vi "Servo MSMT TDSCDMA Create Evaluations.vi"(8 "error in (no error)":errorcluster, 11 "Servo MSMT in":refnum<class "Servo MSMT.lvclass">) -> (0 "error out":errorcluster, 2 "WCDMA Evaluations":T1[](array[typedef]) {"Low Limit" format="%#_13g"; "SI Scaling" items=["femto"=-15, "pico"=-12, "nano"=-9, "micro"=-6, "milli"=-3, "percent"=-2, ""=0, "kilo"=3, "mega"=6, "giga"=9, "tera"=12]}, 3 "Servo MSMT out":refnum<class "Servo MSMT.lvclass">)   [LabVIEW 2018, in "Servo MSMT.lvlib" / "Servo MSMT.lvclass"]
uses:
  Servo MSMT.lvclass
  C:/Sequence Automation/Plugins/Measurement Interface.lvlibp/Measurement Interface.lvclass
  Plugins/TestStand API Tools (TSAT).lvlibp/Evaluation Actions/Includes/Controls/TSAT Evaluation.ctl
  Plugins/TestStand API Tools (TSAT).lvlibp/Evaluation Actions/Includes/Controls/TSAT Eval SI Unit Scaling.ctl
  Plugins/TestStand API Tools (TSAT).lvlibp/Evaluation Actions/Includes/Controls/TSAT Evaluation Type.ctl
  Servo MSMT.lvclass/Servo MSMT.ctl
  Plugins/SeqAuto IEvaluation.lvlibp/SeqAuto IEvaluation.lvclass
  Protected Methods/Read DC Pins.vi
  Protected Methods/Read Servo Measurements.vi
  Plugins/SeqAuto Evaluations.lvlibp/TDSCDMA Evaluations/TDSCDMA_ACP/TDSCDMA_ACP.lvclass
  C:/Sequence Automation/Plugins/SeqAuto IEvaluation.lvlibp/SeqAuto IEvaluation.lvclass
  Plugins/SeqAuto Evaluations.lvlibp/TDSCDMA Evaluations/TDSCDMA_OBW/TDSCDMA_OBW.lvclass
  Plugins/SeqAuto Evaluations.lvlibp/TDSCDMA Evaluations/TDSCDMA_CHP/TDSCDMA_CHP.lvclass
  Plugins/SeqAuto Evaluations.lvlibp/TDSCDMA Evaluations/TDSCDMA_SEM/TDSCDMA_SEM.lvclass
  Plugins/SeqAuto Evaluations.lvlibp/Servo/Servo Gain/Servo Gain.lvclass
  Plugins/SeqAuto Evaluations.lvlibp/PA Evaluations/PAE/PAE.lvclass
  Plugins/SeqAuto Evaluations.lvlibp/TDSCDMA Evaluations/TDSCDMA_MODACC/TDSCDMA_MODACC.lvclass
  Plugins/SeqAuto Evaluations.lvlibp/DC Evaluations/DC_IDD.lvclass
  Plugins/Measurement Interface.lvlibp/Private Methods/Measurement Name/Read Measurement Name.vi
  Plugins/Measurement Interface.lvlibp/Private Methods/Measurement Parameters/Read Measurement Parameters.vi
  Plugins/String Database.lvlibp/String Database.lvclass
  Plugins/TestStand API Tools (TSAT).lvlibp/Evaluation Actions/TSAT Evaluation Actions.lvlib
  Plugins/Test Number and Bin Generator.lvlibp/Test Number and Bin Generator/Test Number and Bin Generator.lvclass
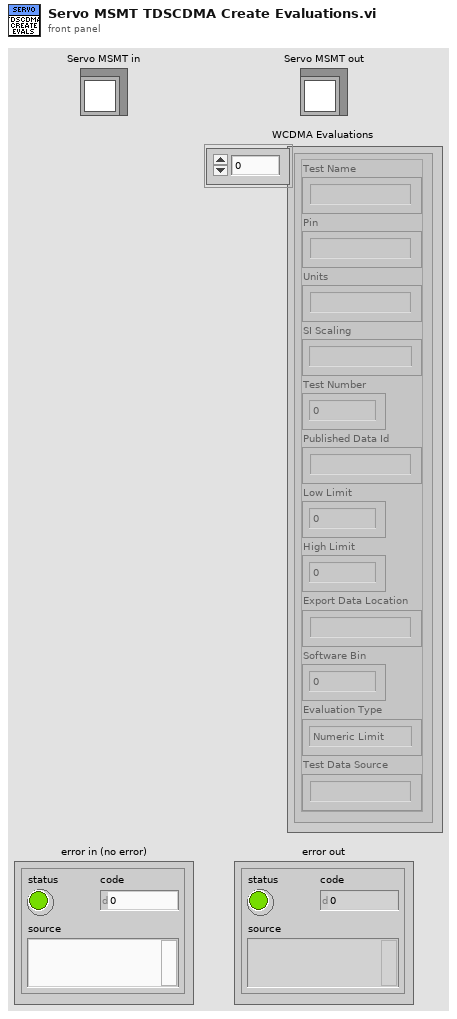
[diagram p1: front panel]
types:
  T1 = typedef "TestStand API Tools (TSAT).lvlibp/TSAT Evaluation Actions.lvlib/TSAT Evaluation.ctl" = cluster{"Test Name":string, "Pin":string, "Units":string, "SI Scaling":T2, "Test Number":i32, "Published Data Id":string, "Low Limit":dbl, "High Limit":dbl, "Export Data Location":string, "Software Bin":i64, "Evaluation Type":T3, "Test Data Source":string}
  T2 = typedef "TestStand API Tools (TSAT).lvlibp/TSAT Evaluation Actions.lvlib/TSAT Eval SI Unit Scaling.ctl" = i16
  T3 = typedef "TestStand API Tools (TSAT).lvlibp/TSAT Evaluation Actions.lvlib/TSAT Evaluation Type.ctl" = enum16{"Numeric Limit", "Pass/Fail", "None"}
  T4 = typedef "Test Number and Bin Generator.lvlibp/Test Number and Bin Generator.lvclass/Session Handle.ctl" = refnum<data-value>
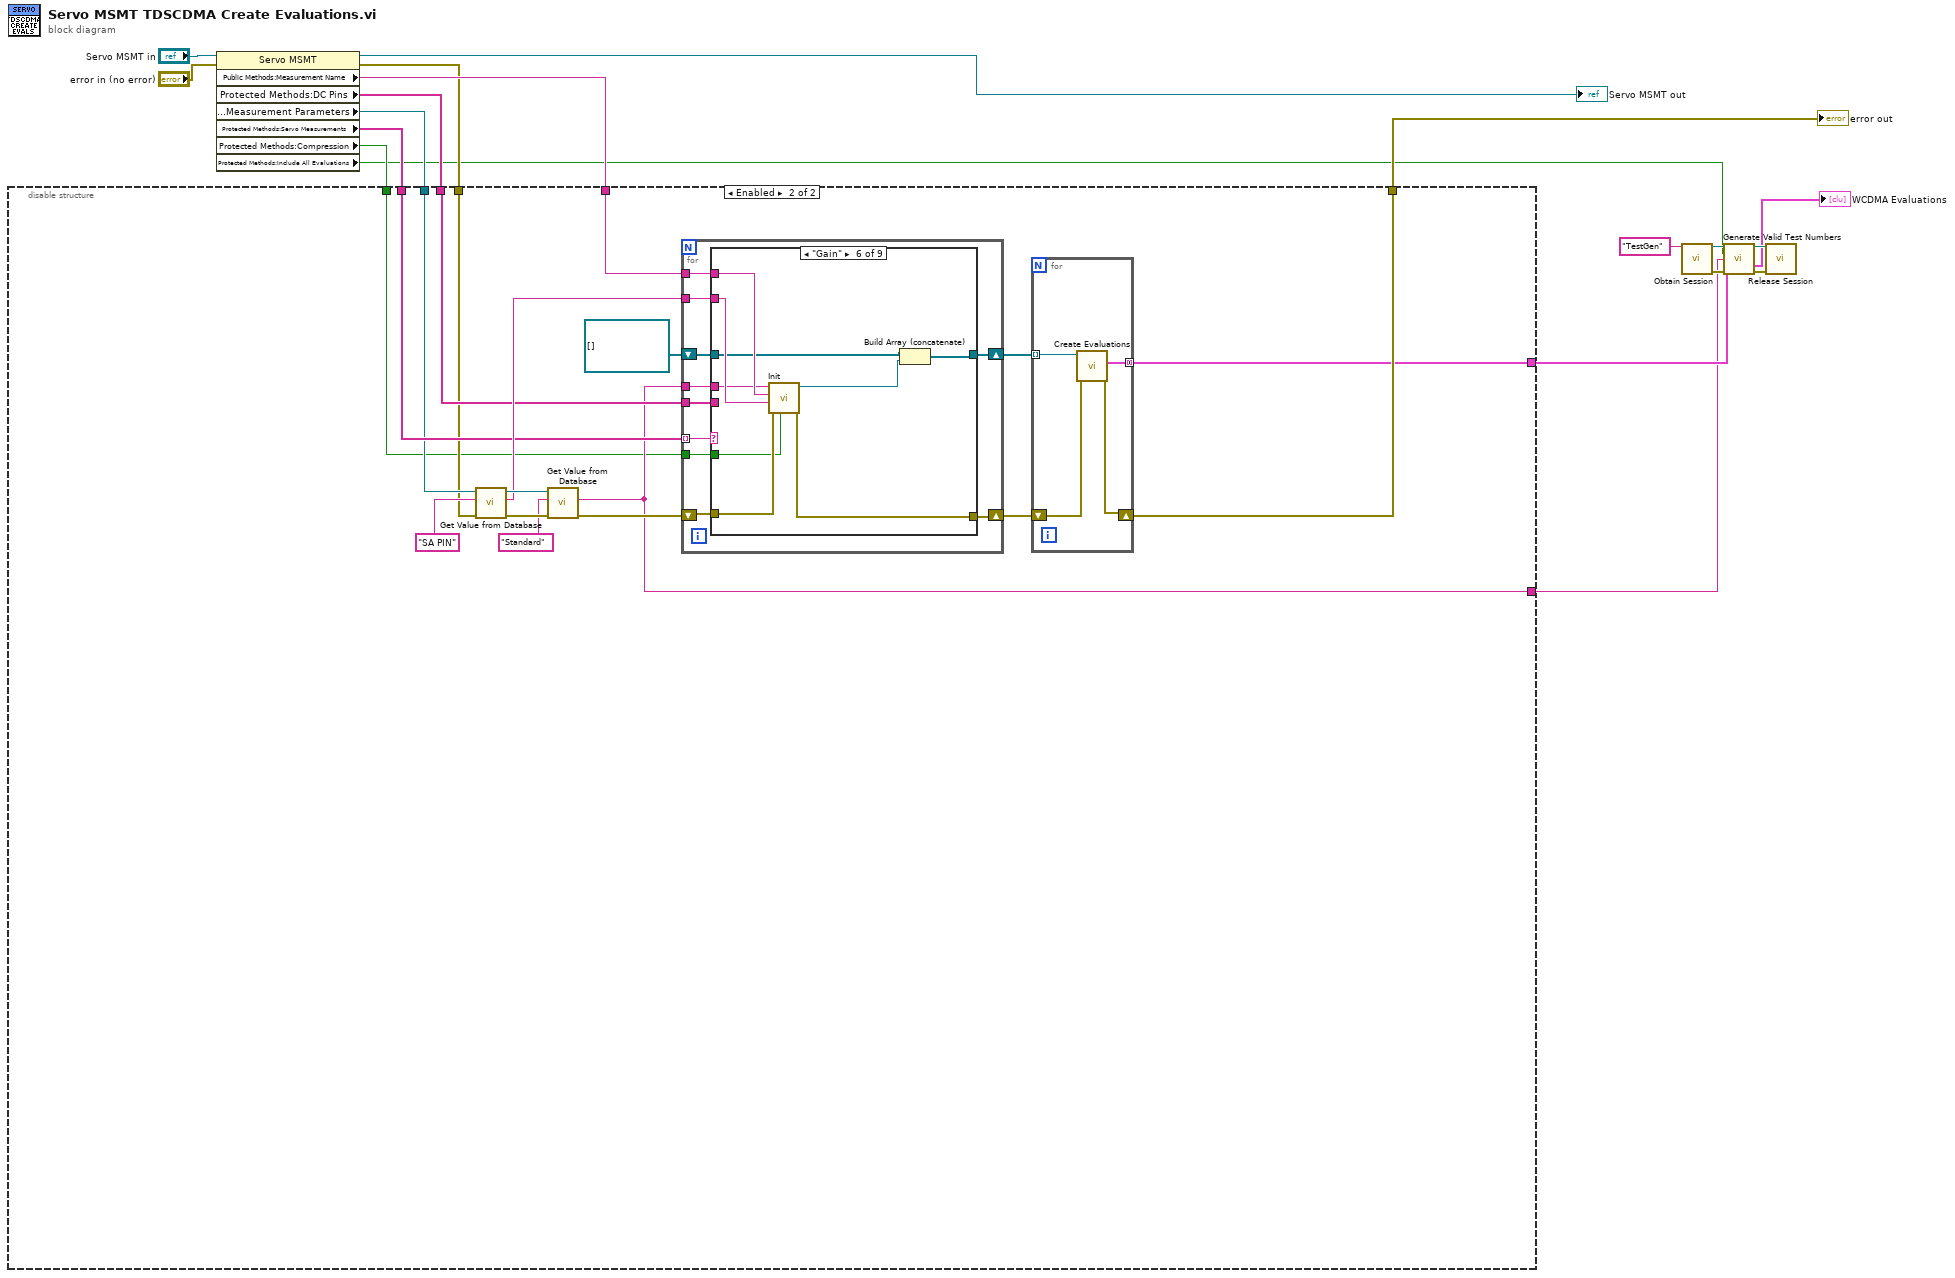
[diagram p0: block diagram]
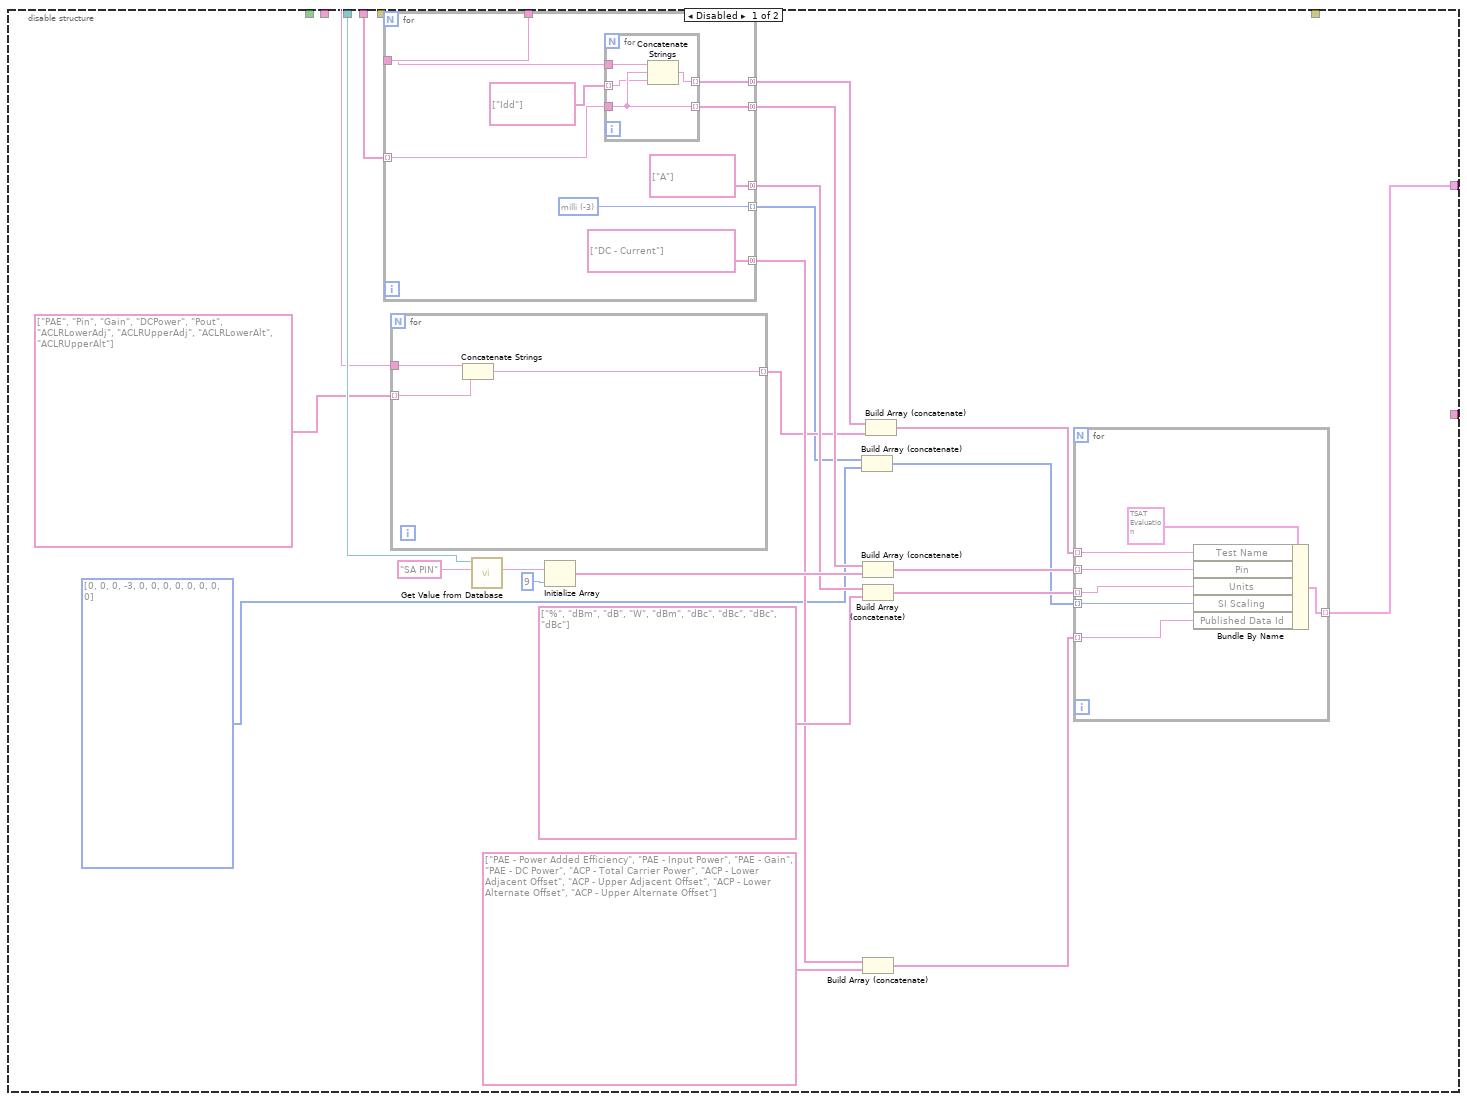
[diagram p2: hidden frame]
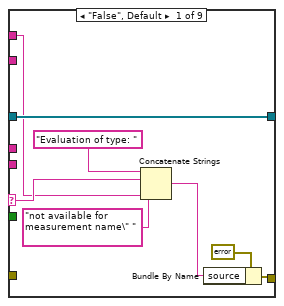
[diagram p3: hidden frame]
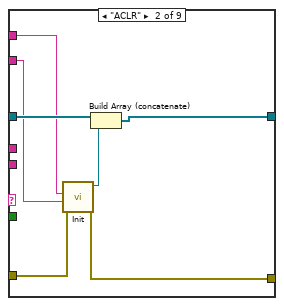
[diagram p4: hidden frame]
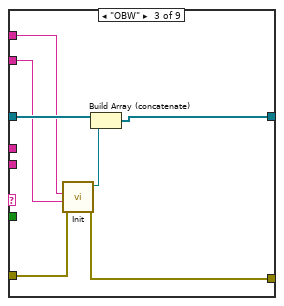
[diagram p5: hidden frame]
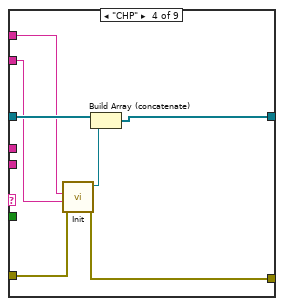
[diagram p6: hidden frame]
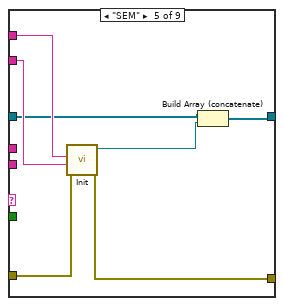
[diagram p7: hidden frame]
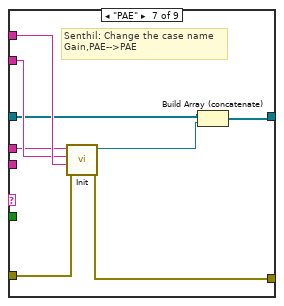
[diagram p8: hidden frame]
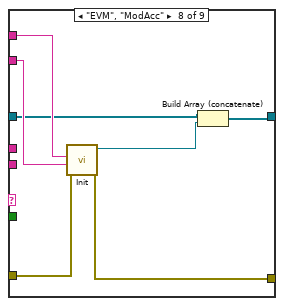
[diagram p9: hidden frame]
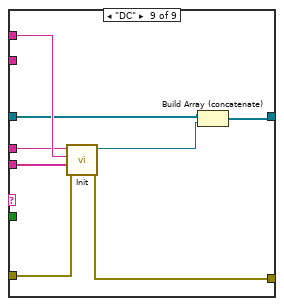
[diagram p10: hidden frame]
diagram:
  n1 = property class="Servo MSMT"(reference="Servo MSMT in", error in="error in (no error)") -> (reference out=→"Servo MSMT out":refnum<class "Servo MSMT.lvclass">, error out=w6:errorcluster, "Public Methods:Measurement Name"=w13:string, "Protected Methods:DC Pins"=w16:string[], "Protected Methods:Measurement Parameters"=w15:refnum<class "String Database.lvclass">, "Protected Methods:Servo Measurements"=w4:string[], "Protected Methods:Compression"=w2:bool, "Protected Methods:Include All Evaluations"=w1:bool)
  n2 = disable-structure shown="Enabled" {
    disable-tunnel: w16 -> [w42 w70]
    disable-tunnel: w15 -> [w40 w71]
    disable-tunnel: w13 -> [w25 w73]
    disable-tunnel: [w20 w66] -> w7
    disable-tunnel: w6 -> [_ w69]
    disable-tunnel: [_ w67] -> w5
    disable-tunnel: w4 -> [_ w72]
    disable-tunnel: [_ w68] -> w3
    disable-tunnel: w2 -> [_ w65]
    frame Disabled {
      w21 = T2[] [0, 0, 0, -3, 0, 0, 0, 0, 0, 0, 0, 0] items=["femto"=-15, "pico"=-12, "nano"=-9, "micro"=-6, "milli"=-3, "percent"=-2, ""=0, "kilo"=3, "mega"=6, "giga"=9, "tera"=12]
      n3 = for {
        tunnel: w42 -> [w50] mode=indexing
        tunnel: w25 -> [w47]
        tunnel: [w52] -> w41 mode=concatenating
        tunnel: [string[] ["A"]] -> w32 mode=concatenating
        tunnel: [w49] -> w36 mode=concatenating
        tunnel: [string[] ["DC - Current"]] -> w30 mode=concatenating
        tunnel: [w46] -> w23 mode=indexing
        w46 = T2 -3 items=["femto"=-15, "pico"=-12, "nano"=-9, "micro"=-6, "milli"=-3, "percent"=-2, ""=0, "kilo"=3, "mega"=6, "giga"=9, "tera"=12] ("SI Scaling")
        n4 = for {
          tunnel: w47 -> [w57]
          tunnel: string[] ["Idd"] -> [w54] mode=indexing
          tunnel: [w56] -> w52 mode=indexing
          tunnel: w50 -> [w55]
          tunnel: [w55] -> w49 mode=indexing
          n5 = Concatenate Strings(w57, w55, w54) -> (w56:string)
        }
      }
      n6 = for {
        tunnel: string[] ["PAE", "Pin", "Gain", "DCPower", "Pout", "ACLRLowerAdj", "ACLRUpperAdj", "ACLRLowerAlt", "ACLRUpperAlt"] -> [w44] mode=indexing
        tunnel: w25 -> [w45]
        tunnel: [w43] -> w24 mode=indexing
        n7 = Concatenate Strings(w45, w44) -> (w43:string)
      }
      n8 = call "Get Value from Database.vi"("Entry Name"="SA PIN", "Message in"=w40) -> ("Entry Value"=w37:string)  [unwired: 6 in, 3 out]
      n9 = Initialize Array(w37, 9) -> (w35:string[])
      n10 = Build Array (concatenate)(w23, w21) -> (w22:T2[])
      n11 = Build Array (concatenate)(w36, w35) -> (w34:string[])
      n12 = Build Array (concatenate)(w32, string[] ["%", "dBm", "dB", "W", "dBm", "dBc", "dBc", "dBc", "dBc"]) -> (w31:string[])
      n13 = Build Array (concatenate)(w30, string[] ["PAE - Power Added Efficiency", "PAE - Input Power", "PAE - Gain", "PAE - DC Power", "ACP - Total Carrier Power", "ACP - Lower Adjacent Offset", "ACP - Upper Adjacent Offset", "ACP - Lower Alternate Offset", "ACP - Upper Alternate Offset"]) -> (w28:string[])
      n14 = Build Array (concatenate)(w41, w24) -> (w27:string[])
      n15 = for {
        tunnel: w27 -> [w63] mode=indexing
        tunnel: [w62] -> w20 mode=indexing
        tunnel: w34 -> [w61] mode=indexing
        tunnel: w31 -> [w60] mode=indexing
        tunnel: w28 -> [w59] mode=indexing
        tunnel: w22 -> [w58] mode=indexing
        n16 = Bundle By Name(cluster=T1 {"Test Name"="test", "Pin"="test", "Units"="dB", "SI Scaling"=-9, "Test Number"=0, "Published Data Id"="test", "Low Limit"=-999999.0, "High Limit"=999999.0, "Export Data Location"="", "Software Bin"=-1, "Evaluation Type"=enum."Numeric Limit", "Test Data Source"=""} ("Evaluation"), "Test Name"=w63, "Pin"=w61, "Units"=w60, "SI Scaling"=w58, "Published Data Id"=w59) -> (w62:T1)
      }
    }
    frame Enabled {
      n17 = call "Get Value from Database.vi"("error in (no error)"=w69, "Entry Name"="SA PIN", "Message in"=w71) -> ("error out"=w81:errorcluster, "Entry Value"=w75:string, "Message out"=w80:refnum<class "String Database.lvclass">)  [unwired: 5 in, 1 out]
      n18 = call "Get Value from Database.vi"("error in (no error)"=w81, "Entry Name"="Standard", "Message in"=w80) -> ("error out"=w74:errorcluster, "Entry Value"=w68:string)  [unwired: 5 in, 2 out]
      n19 = for {
        tunnel: w75 -> [w96]
        tunnel: w73 -> [w95]
        shift-right: [w93] -> w78
        shift-left: refnum<class "SeqAuto IEvaluation.lvclass">[] [] -> [w94]
        tunnel: w72 -> [w92] mode=indexing
        shift-right: [w90] -> w76
        shift-left: w74 -> [w91]
        tunnel: w70 -> [w89]
        tunnel: w68 -> [w88]
        tunnel: w65 -> [w87]
        n20 = case shown="\"Gain\"" w92 {
          selector: w92 -> [w100 _ _ _ _ _ _ _ _]
          tunnel: w96 -> [_ w105 w112 w119 w131 w140 w148 w155 _]
          tunnel: w95 -> [w98 w106 w113 w120 w132 w141 w149 w156 w164]
          tunnel: [w104 w111 w118 w125 w126 w135 w143 w150 w159] -> w93
          tunnel: w94 -> [w104 w110 w117 w124 w128 w137 w145 w152 w161]
          tunnel: w91 -> [_ w108 w115 w122 w130 w139 w147 w154 w163]
          tunnel: [w102 w107 w114 w121 w129 w138 w146 w153 w162] -> w90
          tunnel: w89 -> [_ _ _ _ _ _ _ _ w158]
          tunnel: w88 -> [_ _ _ _ _ w134 w142 _ w157]
          tunnel: w87 -> [_ _ _ _ _ w133 _ _ _]
          frame "False", Default {
            n21 = Concatenate Strings("Evaluation of type: " ("source"), w100, "not available for measurement name\" " ("source"), w98) -> (w97:string)
            n22 = Bundle By Name(cluster=errorcluster {"status"=TRUE, "code"=7777, "source"=""} ("error out"), "source"=w97) -> (w102:errorcluster)
          }
          frame "ACLR" {
            n23 = call "Init.vi"("error in (no error)"=w108, "SA Pin"=w105, "Measurement Name"=w106) -> ("error out"=w107:errorcluster, "TDSCDMA_ACP out"=w109:refnum<class "TDSCDMA_ACP.lvclass">)  [unwired: 7 in]
            n24 = Build Array (concatenate)(w110, w109) -> (w111:refnum<class "SeqAuto IEvaluation.lvclass">[])
          }
          frame "OBW" {
            n25 = call "Init.vi"("error in (no error)"=w115, "SA Pin"=w112, "Measurement Name"=w113) -> ("error out"=w114:errorcluster, "TDSCDMA_OBW out"=w116:refnum<class "TDSCDMA_OBW.lvclass">)  [unwired: 7 in]
            n26 = Build Array (concatenate)(w117, w116) -> (w118:refnum<class "SeqAuto IEvaluation.lvclass">[])
          }
          frame "CHP" {
            n27 = call "Init.vi"("error in (no error)"=w122, "SA Pin"=w119, "Measurement Name"=w120) -> ("error out"=w121:errorcluster, "TDSCDMA_CHP out"=w123:refnum<class "TDSCDMA_CHP.lvclass">)  [unwired: 7 in]
            n28 = Build Array (concatenate)(w124, w123) -> (w125:refnum<class "SeqAuto IEvaluation.lvclass">[])
          }
          frame "SEM" {
            n29 = call "Init.vi"("error in (no error)"=w130, "SA Pin"=w131, "Measurement Name"=w132) -> ("error out"=w129:errorcluster, "TDSCDMA_SEM out"=w127:refnum<class "TDSCDMA_SEM.lvclass">)  [unwired: 7 in]
            n30 = Build Array (concatenate)(w128, w127) -> (w126:refnum<class "SeqAuto IEvaluation.lvclass">[])
          }
          frame "Gain" {
            n31 = call "Init.vi"("Compression?"=w133, "error in (no error)"=w139, "SA Pin"=w140, "Measurement Name"=w141, "Standard"=w134) -> ("error out"=w138:errorcluster, "Servo Gain out"=w136:refnum<class "Servo Gain.lvclass">)  [unwired: 5 in]
            n32 = Build Array (concatenate)(w137, w136) -> (w135:refnum<class "SeqAuto IEvaluation.lvclass">[])
          }
          frame "PAE" {
            # "Senthil: Change the case name\nGain,PAE-->PAE"
            n33 = call "Init.vi"("error in (no error)"=w147, "Measurement Name"=w149, "SA Pin"=w148, "Standard"=w142) -> ("error out"=w146:errorcluster, "PAE out"=w144:refnum<class "PAE.lvclass">)  [unwired: 6 in]
            n34 = Build Array (concatenate)(w145, w144) -> (w143:refnum<class "SeqAuto IEvaluation.lvclass">[])
          }
          frame "EVM", "ModAcc" {
            n35 = call "Init.vi"("error in (no error)"=w154, "SA Pin"=w155, "Measurement Name"=w156) -> ("error out"=w153:errorcluster, "TDSCDMA_MODACC out"=w151:refnum<class "TDSCDMA_MODACC.lvclass">)  [unwired: 7 in]
            n36 = Build Array (concatenate)(w152, w151) -> (w150:refnum<class "SeqAuto IEvaluation.lvclass">[])
          }
          frame "DC" {
            n37 = call "Init.vi"("error in (no error)"=w163, "DC Pins"=w158, "Measurement Name"=w164, "Standard"=w157) -> ("error out"=w162:errorcluster, "DC_IDD out"=w160:refnum<class "DC_IDD.lvclass">)  [unwired: 6 in]
            n38 = Build Array (concatenate)(w161, w160) -> (w159:refnum<class "SeqAuto IEvaluation.lvclass">[])
          }
        }
      }
      n39 = for {
        tunnel: w78 -> [w86] mode=indexing
        tunnel: [w85] -> w66 mode=concatenating
        shift-right: [w83] -> w67
        shift-left: w76 -> [w84]
        n40 = call-dynamic "Create Evaluations.vi"("error in (no error)"=w84, "IEvaluation in"=w86) -> ("error out"=w83:errorcluster, "Evaluations Out"=w85:T1[])  [unwired: 7 in, 1 out]
      }
    }
  }
  "error out" <- w5
  n41 = call "Obtain Session.vi"("Session  Name ()"="TestGen") -> ("Session Handle"=w12:T4, "error out"=w10:errorcluster)  [unwired: 13 in]
  n42 = call "Generate Valid Test Numbers.vi"("Session Handle in"=w12, "Include All Evaluations?"=w1, "Test Group"=w3, "Evaluations In"=w7, "error in (no error)"=w10) -> ("Session Handle out"=w11:T4, "Evaluations Out"=→"WCDMA Evaluations":T1[], "error out"=w9:errorcluster)  [unwired: 8 in]
  n43 = call "Release Session.vi"("Session Handle"=w11, "error in (no error)"=w9) -> ()  [unwired: 13 in, 1 out]
